vi "LtaParseArg.vi"(8 "Error In":errorcluster[](array[cluster]), 10 "Arg In":string="doe1.ray.mi") -> (0 "Error Out":errorcluster[](array[cluster]), 1 "ArgRemaining":string="ray.mi", 2 "Arg 1":string="doe", 3 "Arg1Num":i32=1)   [LabVIEW 2014, in "LTA.lvlib"]
doc: "Arg In: Format Arg[Num].Arg.Arg delimited by \".\"\nArg1Num: [Num] or -1 if there is no [Num]\nArg1 : First Arg with [Num] removed\nArgRemaining: Remaining Args after first Arg[Num] and first delimiting \".\" is removed."
uses:
  LTA.lvlib
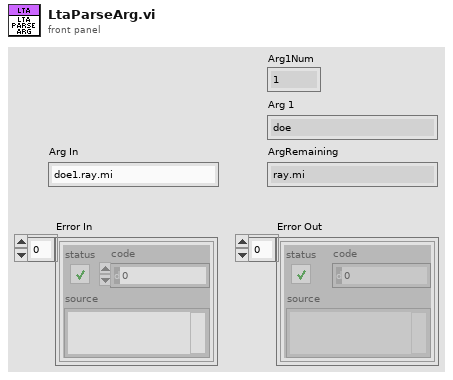
[diagram p1: front panel]
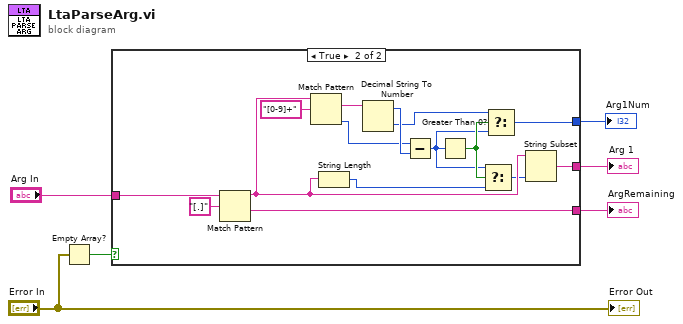
[diagram p0: block diagram]
diagram:
  n1 = Empty Array?(array="Error In") -> (empty?=w6:bool)
  n2 = case shown="True" w6 {
    tunnel: "Arg In" -> [_ w21]
    tunnel: [_ w14] -> w4
    tunnel: [_ w19] -> w3
    tunnel: [_ w7] -> w2
    frame False {
    }
    frame True {
      n3 = Match Pattern(string=w21, regular expression="[.]") -> (before substring=w13:string, after substring=w19:string)  [unwired: 1 in, 2 out]
      n4 = Match Pattern(string=w13, regular expression="[0-9]+") -> (match substring=w17:string, offset past match=w15:i32)  [unwired: 1 in, 2 out]
      n5 = String Length(string=w13) -> (length=w11:i32)
      n6 = Decimal String To Number(string=w17) -> (offset past number=w16:i32, number=w9:i32)  [unwired: 2 in]
      n7 = Subtract(x=w15, y=w16) -> (x-y=w8:i32)
      n8 = Greater Than 0?(x=w8) -> (x > 0?=w10:bool)
      n9 = Select(t=w8, s=w10, f=w11) -> (s? t:f=w12:i32)
      n10 = Select(t=w9, s=w10, f=w8) -> (s? t:f=w7:i32)
      n11 = String Subset(string=w13, length (rest)=w12) -> (substring=w14:string)  [unwired: 1 in]
    }
  }
  "Arg 1" <- w4
  "ArgRemaining" <- w3
  "Arg1Num" <- w2
  "Error Out" <- "Error In"
